vi "Unpacked KM Data to FIFO.vi"(9 "output valid?":bool, 10 "Unpacked data":u32, 11 "Num of data in":u32) -> (2 "in time":bool, 3 "Num of data out":u32)   [LabVIEW 2015]
uses:
  <vilib>/rvi/interface/RandomDataEmulation/niFpgaRandomDataHandleErrors.vi
  <vilib>/rvi/DataTransferAndStorage/Container/XNode/niFpgaContainer.xnode
  <vilib>/rvi/interface/RandomDataEmulation/nirviRandomDataFpgaReadWriteTemplate.vi
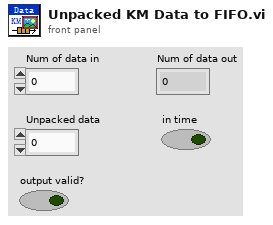
[diagram p1: front panel]
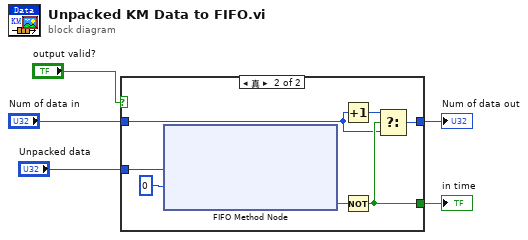
[diagram p0: block diagram]
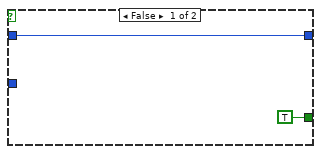
[diagram p2: hidden frame]
diagram:
  n1 = case shown="真" "output valid?" {
    tunnel: [TRUE w11] -> w1
    tunnel: "Num of data in" -> [w6 w10]
    tunnel: [w6 w9] -> w5
    tunnel: "Unpacked data" -> [_ w8]
    frame False {
    }
    frame True {
      n2 = xnode ("FIFO Method Node")("元素"=w8, "超时"=0 ("Timeout")) -> ("超时？"=w13:bool)  [unwired: 1 in, 1 out]
      n3 = Increment(x=w10) -> (x+1=w12:u32)
      n4 = Not(x=w13) -> (.not. x?=w11:bool)
      n5 = Select(t=w12, s=w11, f=w10) -> (s? t:f=w9:u32)
    }
  }
  "Num of data out" <- w5
  "in time" <- w1
